vi "Add Command.vi"(7 "State":string, 8 "error in (no error)":errorcluster, 9 "Command Config":refnum<class "Command Config.lvclass">, 10 "Time":dbl, 11 "Sequence Config in":refnum<class "Sequence Config.lvclass">) -> (0 "error out":errorcluster, 3 "Sequence Config out":refnum<class "Sequence Config.lvclass">)   [LabVIEW 2020, in "VolatusSeqConfig.lvlib" / "Sequence Config.lvclass"]
uses:
  Sequence Config.lvclass
  Sequence Config.lvclass/Sequence Config.ctl
  Command Config/Command Config.lvclass
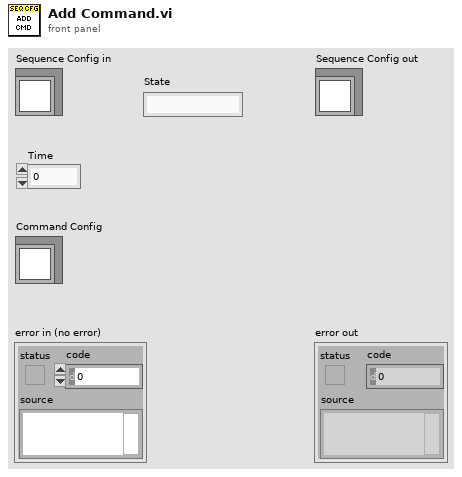
[diagram p1: front panel]
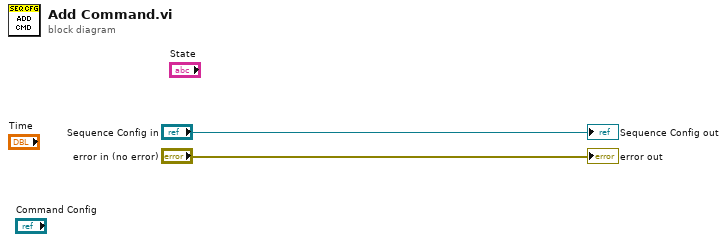
[diagram p0: block diagram]
diagram:
  "error out" <- "error in (no error)"
  "Sequence Config out" <- "Sequence Config in"
